vi "ShutterOpen.vi"(8 "error in (no error)":errorcluster, 10 "Shutter number":i32, 11 "Microscope in":refnum<class "Microscope.lvclass">) -> (0 "error out":errorcluster, 3 "Microscope out":refnum<class "Microscope.lvclass">)   [LabVIEW 2012, in "Microscope.lvclass"]
uses:
  classes/Microscope.lvclass
  classes/Microscope.lvclass/Microscope.ctl
  <vilib>/DAQmx/write.llb/DAQmx Write (Digital Bool 1Line 1Point).vi
  <vilib>/DAQmx/create/channels.llb/DAQmx Create Channel (DO-Digital Output).vi
  <vilib>/DAQmx/miscellaneous.llb/DAQmx Fill In Error Info.vi
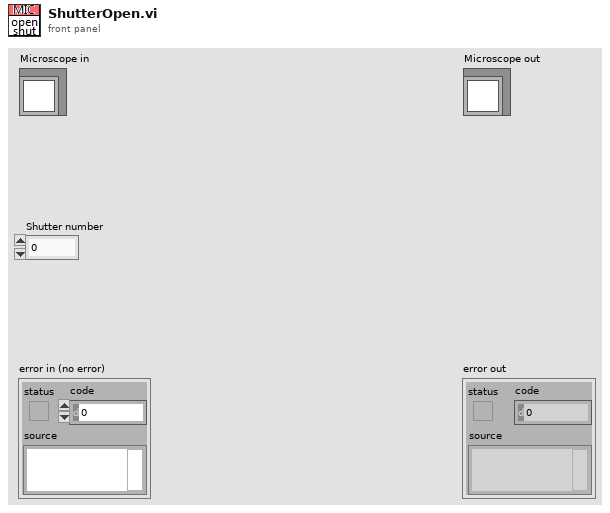
[diagram p1: front panel]
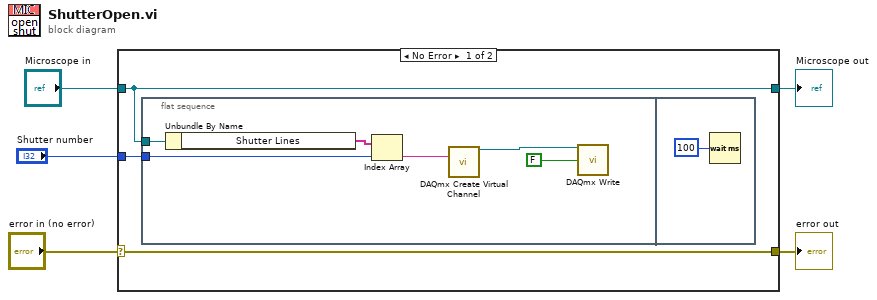
[diagram p0: block diagram]
diagram:
  n1 = case shown="No Error" "error in (no error)" {
    selector: "error in (no error)" -> [w8 w17]
    tunnel: [w8 w17] -> w4
    tunnel: [w6 w16] -> w2
    tunnel: "Microscope in" -> [w6 w16]
    tunnel: "Shutter number" -> [w7 _]
    frame No Error {
      n2 = flat-sequence {
        tunnel: w7 -> [w12]
        tunnel: w6 -> [w9]
        frame #0 {
          n3 = Unbundle By Name(w9) -> ("Shutter Lines"=w13:tag[])
          n4 = Index Array(array=w13, index=w12) -> (element=w11:tag)
          n5 = call-poly <vilib>:"DAQmx Create Virtual Channel.vi"("lines"=w11) -> ("task out"=w10:refnum<k21>)  [unwired: 13 in, 1 out]
          n6 = call-poly <vilib>:"DAQmx Write.vi"("task/channels in"=w10, "data"=FALSE) -> ()  [unwired: 11 in, 3 out]
        }
        frame #1 {
          n7 = Wait (ms)(milliseconds to wait=u32 100) -> ()  [unwired: 1 out]
        }
      }
    }
    frame Error {
    }
  }
  "error out" <- w4
  "Microscope out" <- w2
